vi "Polar_Arrays_To_Chart.vi"(10 "Direction":dbl[](array[numeric]), 11 "Magnitude":dbl[](array[numeric])) -> (3 "Scan":cluster{"x":dbl, "y":dbl}[](array[cluster]))   [LabVIEW 2016]
uses:
  <vilib>/ptbypt/NI_PtbyPt.lvlib
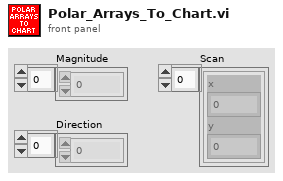
[diagram p1: front panel]
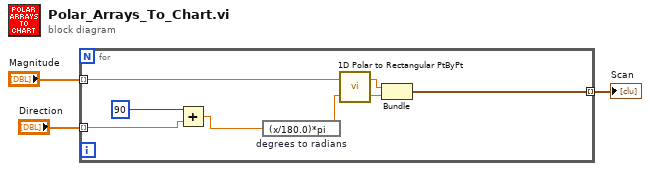
[diagram p0: block diagram]
diagram:
  n1 = for {
    tunnel: "Magnitude" -> [w11] mode=indexing
    tunnel: "Direction" -> [w6] mode=indexing
    tunnel: [w8] -> w3 mode=indexing
    n2 = Add(x=90, y=w6) -> (x+y=w4:dbl)
    n3 = expression code="(x/180.0)*pi" "degrees to radians"(w4) -> (w7:dbl)
    n4 = call <vilib>:"1D Polar to Rectangular PtByPt.vi"("phase"=w7, "magnitude"=w11) -> ("y"=w10:dbl, "x"=w9:dbl)
    n5 = Bundle("x"=w9, "y"=w10) -> (w8:cluster{"x":dbl, "y":dbl})  [unwired: 1 in]
  }
  "Scan" <- w3
